vi "QueueRepo.vi"(7 "Action":T1, 8 "error in (no error)":errorcluster, 9 "Event?":bool, 11 "Name":string) -> (0 "error out":errorcluster, 1 "Event?":bool, 2 "queue out":refnum<queue>, 3 "Names":string[](array[string]))   [LabVIEW 2017, in "Communication.lvlib"]
uses:
  Communication.lvlib
  QueueRepo.Action.ctl
  MsgData.ctl
  MsgAck.ctl
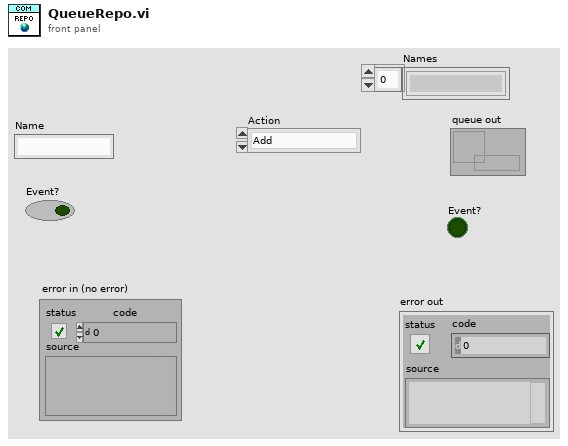
[diagram p1: front panel]
types:
  T1 = typedef "Communication.lvlib/QueueRepo.Action.ctl" = enum16{"Add", "Get", "Destroy", "Get All", "Clear"}
  T2 = typedef "Communication.lvlib/MsgData.ctl" = cluster{"Msg":string, "Data":variant, "Ack":refnum<notifier>}
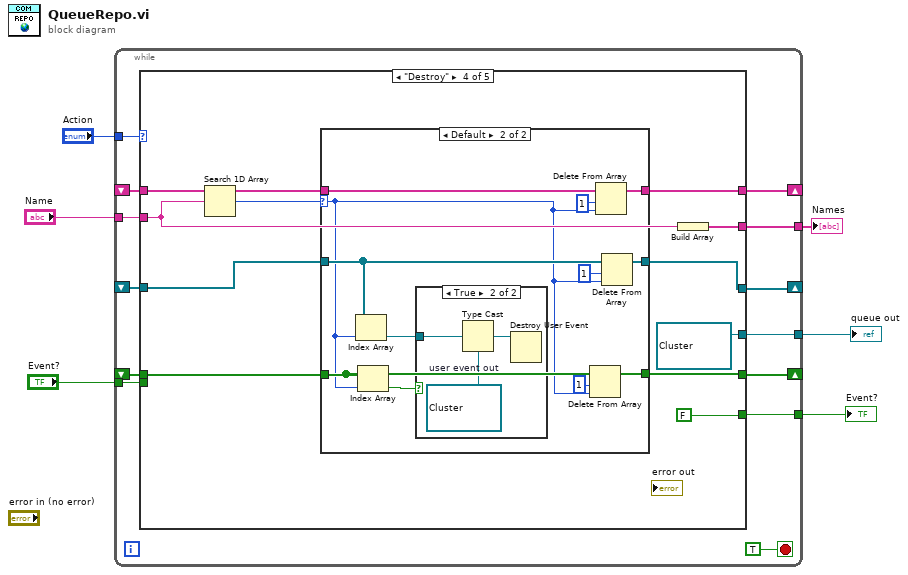
[diagram p0: block diagram]
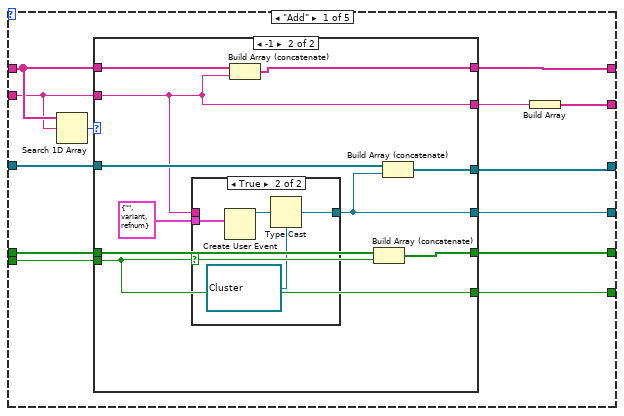
[diagram p2: hidden frame]
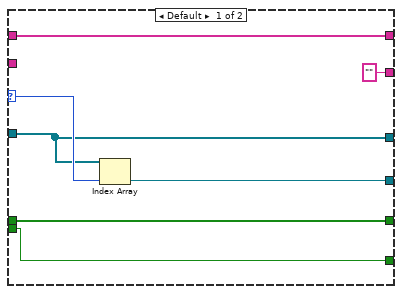
[diagram p3: hidden frame]
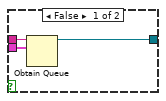
[diagram p4: hidden frame]
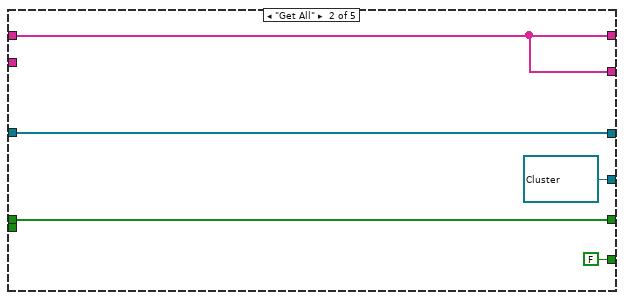
[diagram p5: hidden frame]
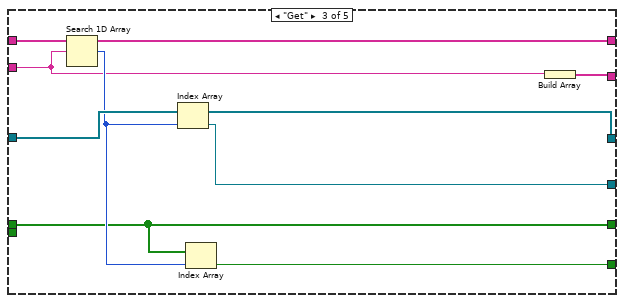
[diagram p6: hidden frame]
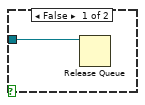
[diagram p8: hidden frame]
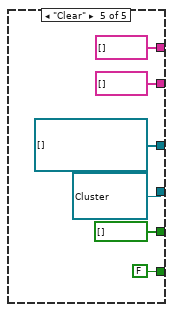
[diagram p9: hidden frame]
diagram:
  n1 = while {
    tunnel: "Action" -> [w19]
    tunnel: "Name" -> [w18]
    shift-right: [w16] -> _
    shift-left: _ -> [w15]
    shift-right: [w14] -> _
    shift-left: _ -> [w13]
    tunnel: [w12] -> w4
    tunnel: "Event?" -> [w11]
    shift-right: [w10] -> _
    shift-left: _ -> [w9]
    tunnel: [w8] -> w2
    tunnel: [w7] -> w1
    stop <- TRUE stop-if-true
    n2 = case shown="\"Destroy\"" w19 {
      tunnel: w18 -> [w30 _ w62 w73 _]
      tunnel: [w32 w60 w67 w70 string[] []] -> w16
      tunnel: w15 -> [w31 w60 w67 w71 _]
      tunnel: [w28 w61 w68 w79 refnum<queue>[] []] -> w14
      tunnel: w13 -> [w27 w61 w68 w80 _]
      tunnel: [w26 refnum<queue> refnum ("queue out") w69 refnum<queue> refnum ("queue out") refnum<queue> refnum ("queue out")] -> w12
      tunnel: w11 -> [w25 _ _ _ _]
      tunnel: [w24 w58 w65 w75 bool[] []] -> w10
      tunnel: w9 -> [w23 w58 w65 w76 _]
      tunnel: [w22 FALSE ("Event?") w64 FALSE FALSE ("Event?")] -> w8
      tunnel: [w20 w60 w63 w72 string[] []] -> w7
      frame "Add" {
        n3 = Search 1D Array(1D array=w31, element=w30) -> (index of element=w29:i32)  [unwired: 1 in]
        n4 = case shown="-1" w29 {
          selector: w29 -> [w38 _]
          tunnel: [w39 w40] -> w32
          tunnel: w31 -> [w39 w49]
          tunnel: w30 -> [_ w41]
          tunnel: [w37 w47] -> w28
          tunnel: w27 -> [w37 w46]
          tunnel: [w36 w45] -> w26
          tunnel: w25 -> [w35 w42]
          tunnel: [w34 w44] -> w24
          tunnel: w23 -> [w34 w43]
          tunnel: [w35 w42] -> w22
          tunnel: ["" ("Name") w41] -> w21
          frame Default {
            n5 = Index Array(array=w37, index=w38) -> (element=w36:refnum<queue>)
          }
          frame -1 {
            n6 = case shown="True" w42 {
              tunnel: w41 -> [w52 _]
              tunnel: T2 {"Msg"="", "Data"=variant, "Ack"=refnum} ("Cluster") -> [w51 w56]
              tunnel: [w50 w53] -> w45
              frame False {
                n7 = Obtain Queue(name (unnamed)=w52, element data type=w51) -> (queue out=w50:refnum<queue>)  [unwired: 3 in, 2 out]
              }
              frame True {
                n8 = Create User Event(user event datatype=w56) -> (user event=w55:refnum<user-event>)  [unwired: 1 in, 1 out]
                n9 = Type Cast(type=refnum<queue> refnum ("queue out"), x=w55) -> (*(type *) &x=w53:refnum<queue>)
              }
            }
            n10 = Build Array (concatenate)(w49, w41) -> (w40:string[])
            n11 = Build Array (concatenate)(w43, w42) -> (w44:bool[])
            n12 = Build Array (concatenate)(w46, w45) -> (w47:refnum<queue>[])
          }
        }
        n13 = Build Array(w21) -> (w20:string[])
      }
      frame "Get All" {
      }
      frame "Get" {
        n14 = Search 1D Array(1D array=w67, element=w62) -> (index of element=w66:i32)  [unwired: 1 in]
        n15 = Index Array(array=w68, index=w66) -> (element=w69:refnum<queue>)
        n16 = Index Array(array=w65, index=w66) -> (element=w64:bool)
        n17 = Build Array(w62) -> (w63:string[])
      }
      frame "Destroy" {
        n18 = Search 1D Array(1D array=w71, element=w73) -> (index of element=w77:i32)  [unwired: 1 in]
        n19 = case shown="Default" w77 {
          selector: w77 -> [_ w84]
          tunnel: w80 -> [w83 w94]
          tunnel: [w83 w93] -> w79
          tunnel: w76 -> [w82 w90]
          tunnel: [w82 w89] -> w75
          tunnel: w71 -> [w81 w87]
          tunnel: [w81 w86] -> w70
          frame -1 {
          }
          frame Default {
            n20 = Index Array(array=w94, index=w84) -> (element=w95:refnum<queue>)
            n21 = Index Array(array=w90, index=w84) -> (element=w91:bool)
            n22 = case shown="True" w91 {
              tunnel: w95 -> [w96 w99]
              frame False {
                n23 = Release Queue(queue=w96) -> ()  [unwired: 2 in, 3 out]
              }
              frame True {
                w98 = refnum<user-event> refnum  # user event out
                n24 = Type Cast(type=w98, x=w99) -> (*(type *) &x=w97:refnum<user-event>)
                n25 = Destroy User Event(user event=w97) -> ()  [unwired: 1 in, 1 out]
              }
            }
            n26 = Delete From Array(array=w90, length=1, index=w84) -> (array with subset deleted=w89:bool[])  [unwired: 1 out]
            n27 = Delete From Array(array=w87, length=1, index=w84) -> (array with subset deleted=w86:string[])  [unwired: 1 out]
            n28 = Delete From Array(array=w94, length=1, index=w84) -> (array with subset deleted=w93:refnum<queue>[])  [unwired: 1 out]
          }
        }
        n29 = Build Array(w73) -> (w72:string[])
      }
      frame "Clear" {
      }
    }
  }
  "queue out" <- w4
  "Event?" <- w2
  "Names" <- w1
